vi "256_to_10.vi"(1 "Array":i32[](array[numeric])) -> (0 "Numeric":dbl)   [LabVIEW 2015, in "PolyVIEW.lvclass"]
uses:
  PolyVIEW.lvclass
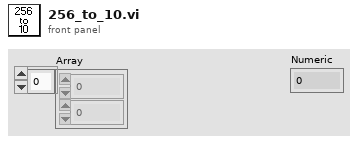
[diagram p1: front panel]
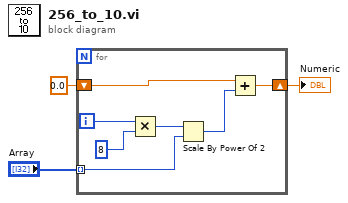
[diagram p0: block diagram]
diagram:
  n1 = for {
    tunnel: "Array" -> [w5] mode=indexing
    shift-right: [w10] -> w1
    shift-left: 0.0 -> [w9]
    i -> [w7]
    n2 = Multiply(x=w7, y=8) -> (x*y=w6:i32)
    n3 = Scale By Power Of 2(n=w6, x=w5) -> (x*2^n=w4:i32)
    n4 = Add(x=w9, y=w4) -> (x+y=w10:dbl)
  }
  "Numeric" <- w1
